vi "SwerveChooseAngle.vi"() -> ()   [LabVIEW 2018]
panel:
  out "Distance to Goal":dbl
  out "Boolean Flag":dbl
  out "Chosen Goal Angle":dbl
  in  "Joystick Goal Angle":dbl
  in  "Current Angle":dbl
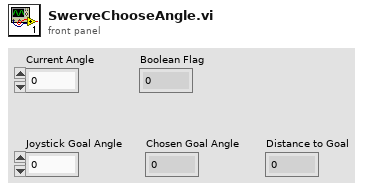
[diagram p1: front panel]
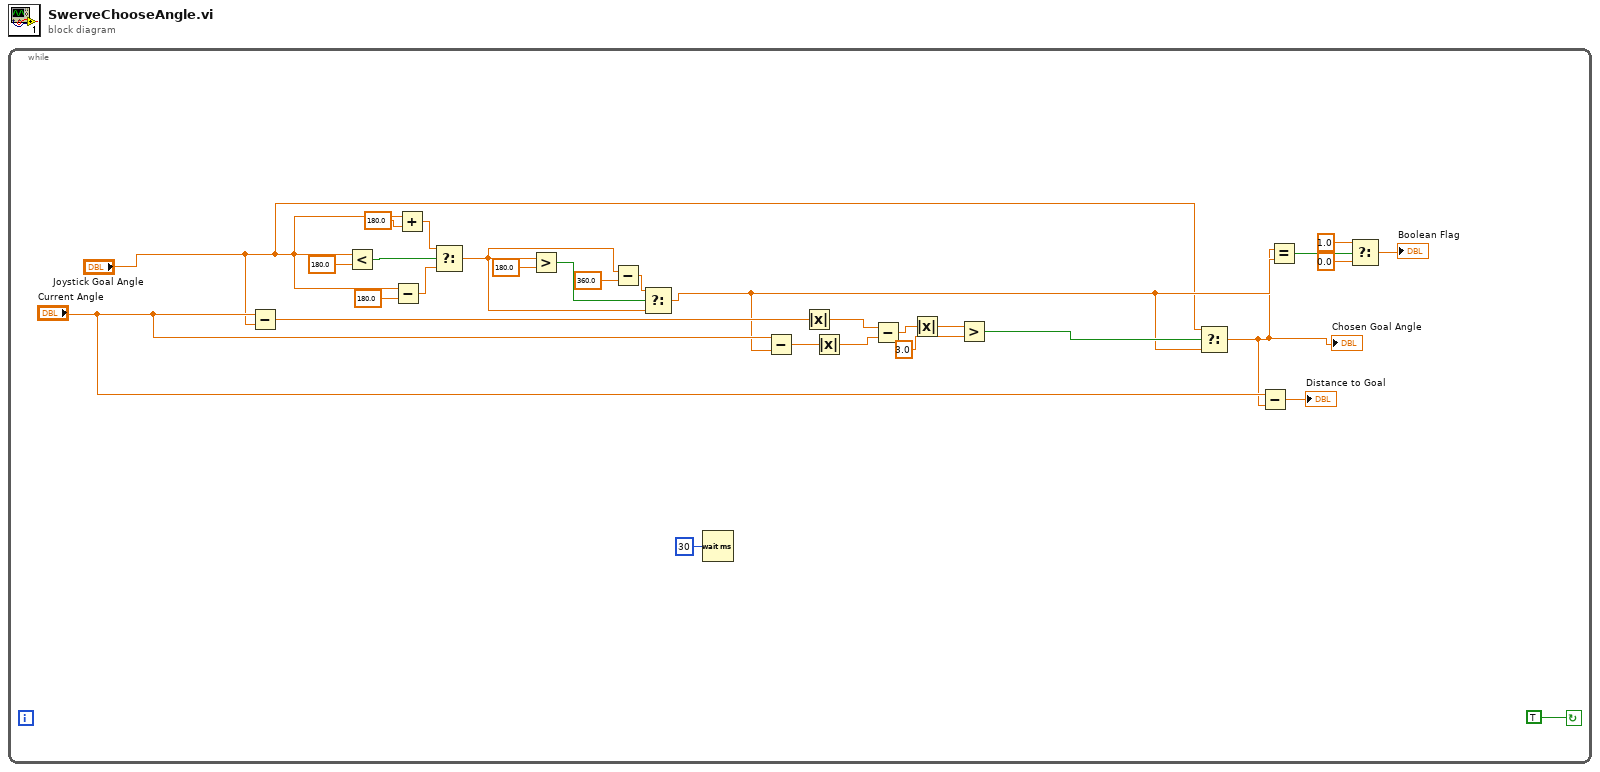
[diagram p0: block diagram]
diagram:
  n1 = while {
    stop <- TRUE continue-if-true
    n2 = Subtract(x="Current Angle", y="Joystick Goal Angle") -> (x-y=w24:dbl)
    n3 = Less?(x="Joystick Goal Angle", y=180.0) -> (x < y?=w29:bool)
    n4 = Subtract(x="Joystick Goal Angle", y=180.0) -> (x-y=w26:dbl)
    n5 = Add(x="Joystick Goal Angle", y=180.0) -> (x+y=w27:dbl)
    n6 = Select(t=w27, s=w29, f=w26) -> (s? t:f=w10:dbl)
    n7 = Greater?(x=w10, y=180.0) -> (0:w13:bool)
    n8 = Subtract(x=w10, y=360.0) -> (x-y=w15:dbl)
    n9 = Select(t=w15, s=w13, f=w10) -> (s? t:f=w12:dbl)
    n10 = Wait (ms)(milliseconds to wait=u32 30) -> ()  [unwired: 1 out]
    n11 = Subtract(x="Current Angle", y=w12) -> (x-y=w22:dbl)
    n12 = Absolute Value(x=w24) -> (abs(x)=w6:dbl)
    n13 = Absolute Value(x=w22) -> (abs(x)=w5:dbl)
    n14 = Subtract(x=w6, y=w5) -> (x-y=w3:dbl)
    n15 = Absolute Value(x=w3) -> (abs(x)=w1:dbl)
    n16 = Greater?(x=w1, y=3.0) -> (0:w23:bool)
    n17 = Select(t="Joystick Goal Angle", s=w23, f=w12) -> (s? t:f=w2:dbl)
    "Chosen Goal Angle" <- w2
    n18 = Subtract(x="Current Angle", y=w2) -> (x-y=→"Distance to Goal":dbl)
    n19 = Equal?(x=w2, y=w12) -> (x = y?=w21:bool)
    n20 = Select(t=1.0, s=w21, f=0.0) -> (s? t:f=→"Boolean Flag":dbl)
  }
